vi "libssh2_channel_forward_listen_ex.vi"(7 "queue_maxsize":i32, 8 "error in (no error)":errorcluster, 9 "port":i32, 10 "host":string, 11 "session":u64) -> (0 "error out":errorcluster, 2 "bound_port":i32, 3 "return value":u64)   [LabVIEW 2013, in "libssh2.lvlib"]
uses:
  libssh2.lvlib
  libssh2.dll
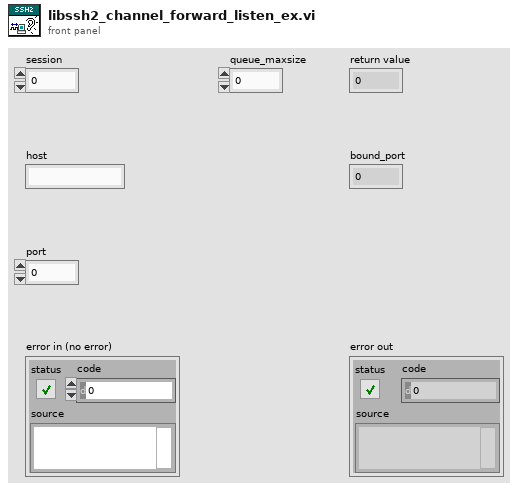
[diagram p1: front panel]
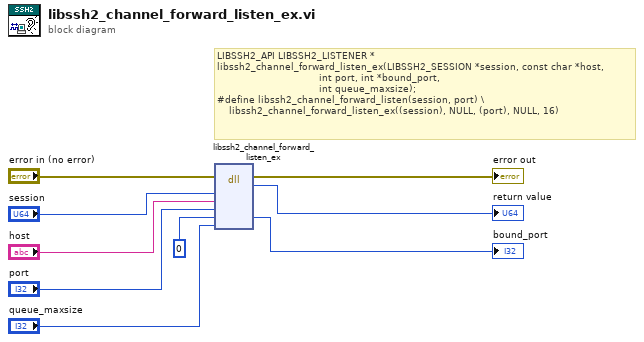
[diagram p0: block diagram]
diagram:
  # "LIBSSH2_API LIBSSH2_LISTENER *\nlibssh2_channel_forward_listen_ex(LIBSSH2_SESSION *session, const char *host,\n                                  int port, int *bound_port,\n                                  int queue_maxsize);\n#define libssh2_channel_forward_listen(session, port) \\\n    libssh2_channel_forward_listen_ex((session), NULL, (port), NULL, 16)"
  n1 = dll-call lib="C:/Users/pasca/source/repos/libssh2-labview/libssh2**.*" fn="libssh2_channel_forward_listen_ex"(error in="error in (no error)", "session"="session", "host"="host", "port"="port", "bound_port"=0, "queue_maxsize"="queue_maxsize") -> (error out=→"error out":errorcluster, "return value"=→"return value":u64, "bound_port"=→"bound_port":i32)  [unwired: 6 in, 1 out]
